vi "A87.6-decoder.vi"(10 "参考电压（V）":dbl=2.56, 11 "编码数组":digitaldata) -> (3 "还原信号数组":dbl[](array[numeric]))   [LabVIEW 2018]
uses:
  <vilib>/Waveform/DTblOps.llb/DTbl Digital to Boolean Array.vi
panel:
  # "输入：编码数组（数字数据），参考电压Vref\n输出：复原信号数组"
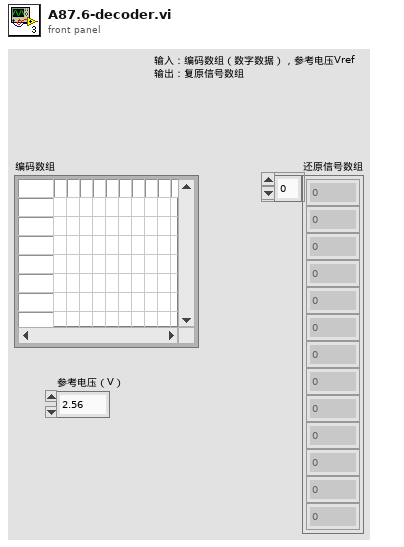
[diagram p1: front panel]
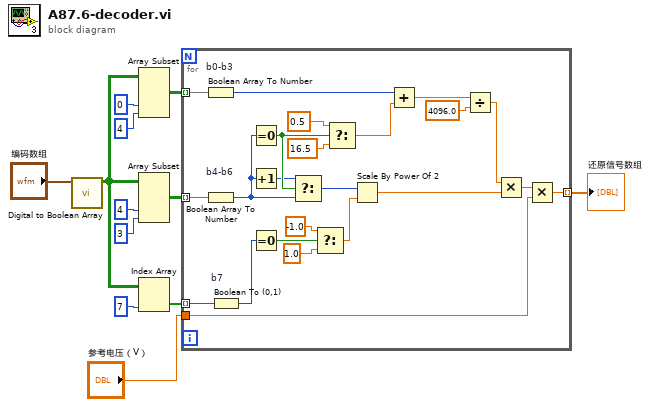
[diagram p0: block diagram]
diagram:
  n1 = call-poly <vilib>:"Digital to Boolean Array.vi"("digital data"="编码数组") -> ("boolean array"=w5:bool[][])  [unwired: 9 in, 1 out]
  n2 = Array Subset(array=w5, index (col)=0 ("索引"), length (col)=4 ("长度")) -> (w9:bool[][])  [unwired: 2 in]
  n3 = Array Subset(array=w5, index (col)=4 ("索引"), length (col)=3 ("长度")) -> (w6:bool[][])  [unwired: 2 in]
  n4 = Index Array(array=w5, index (col)=7 ("禁用的索引 (列)")) -> (element=w3:bool[])  [unwired: 1 in]
  n5 = for {
    tunnel: w9 -> [w35] mode=indexing
    tunnel: w6 -> [w34] mode=indexing
    tunnel: w3 -> [w33] mode=indexing
    tunnel: "参考电压（V）" -> [w14]
    tunnel: [w13] -> w1 mode=indexing
    n6 = Boolean Array To Number "b0-b3"(Boolean array=w35) -> (number=w22:u32)
    n7 = Boolean Array To Number "b4-b6"(Boolean array=w34) -> (number=w31:u32)
    n8 = Boolean To (0,1) "b7"(Boolean=w33) -> (0, 1=w27:i16)
    n9 = Equal To 0?(x=w31) -> (x = 0?=w32:bool)
    n10 = Increment(x=w31) -> (x+1=w30:u32)
    n11 = Equal To 0?(x=w27) -> (x = 0?=w26:bool)
    n12 = Select(t=w30, s=w32, f=w31) -> (s? t:f=w21:u32)
    n13 = Select(t=-1.0, s=w26, f=1.0) -> (s? t:f=w20:dbl)
    n14 = Select(t=0.5, s=w32, f=16.5) -> (s? t:f=w23:dbl)
    n15 = Scale By Power Of 2(n=w21, x=w20) -> (x*2^n=w16:dbl)
    n16 = Add(x=w22, y=w23) -> (x+y=w19:dbl)
    n17 = Divide(x=w19, y=4096.0) -> (x/y=w17:dbl)
    n18 = Multiply(x=w17, y=w16) -> (x*y=w15:dbl)
    n19 = Multiply(x=w15, y=w14) -> (x*y=w13:dbl)
  }
  "还原信号数组" <- w1
